vi "SetG.vi"(8 "error in (no error)":errorcluster, 10 "G":u8, 11 "ColorRGB in":refnum<class "ColorRGB.lvclass">) -> (0 "error out":errorcluster, 3 "ColorRGB out":refnum<class "ColorRGB.lvclass">)   [LabVIEW 2021, in "Picture2D.lvlib" / "ColorRGB.lvclass"]
uses:
  ColorRGB.lvclass
  ColorRGB.lvclass/ColorRGB.ctl
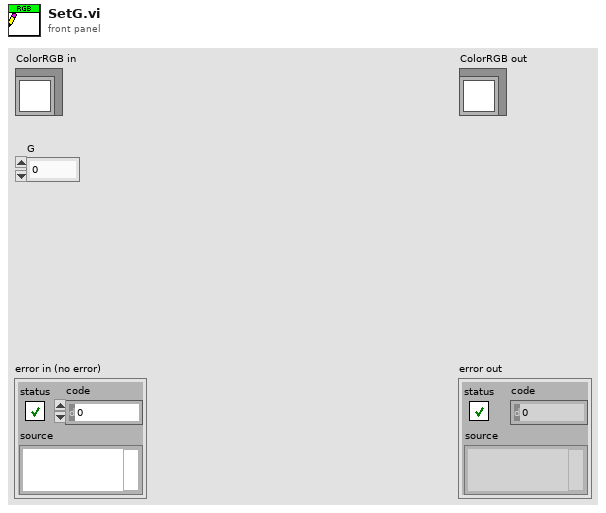
[diagram p1: front panel]
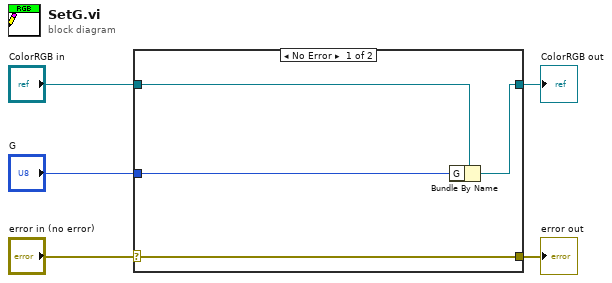
[diagram p0: block diagram]
diagram:
  n1 = case shown="No Error" "error in (no error)" {
    selector: "error in (no error)" -> [w9 w10]
    tunnel: [w9 w10] -> w4
    tunnel: [w7 w11] -> w2
    tunnel: "ColorRGB in" -> [w8 w11]
    tunnel: "G" -> [w6 _]
    frame No Error {
      n2 = Bundle By Name(cluster=w8, "G"=w6) -> (w7:refnum<class "ColorRGB.lvclass">)
    }
    frame Error {
    }
  }
  "error out" <- w4
  "ColorRGB out" <- w2
